vi "FRCts20_Backend_SaveTimer.vi"(8 "error in (no error)":errorcluster, 10 "Data Changed?":bool) -> (0 "error out":errorcluster)   [LabVIEW 2014, in "FRCts20_Backend_Engine.lvlib"]
doc: "This counts the time and if we have reached 5 minutes of idle time and the data changed, we send an AMC command to save everything."
uses:
  FRCts20_Backend_Engine.lvlib
  FRCts20_Backend_FGVOperation.ctl
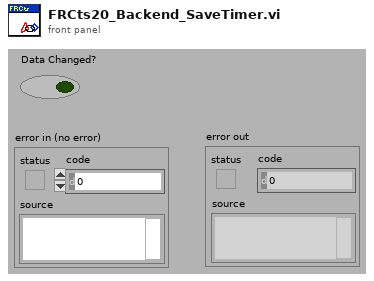
[diagram p1: front panel]
types:
  T1 = typedef "FRCts20_Backend_Engine.lvlib/FRCts20_Backend_FGVOperation.ctl" = enum16{"Initialize", "EnqueueMessage", "EnqueueDataReturn", "FlushMessage", "FlushDataReturn"}
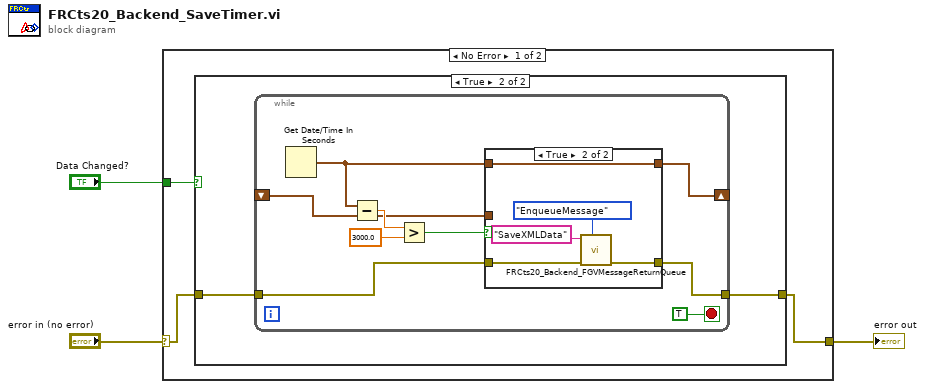
[diagram p0: block diagram]
diagram:
  n1 = case shown="No Error" "error in (no error)" {
    selector: "error in (no error)" -> [w5 w26]
    tunnel: [w4 w26] -> w2
    tunnel: "Data Changed?" -> [w6 _]
    frame No Error {
      n2 = case shown="True" w6 {
        tunnel: w5 -> [w7 w9]
        tunnel: [w7 w8] -> w4
        frame False {
        }
        frame True {
          n3 = while {
            shift-right: [w11] -> _
            shift-left: _ -> [w10]
            tunnel: w9 -> [w14]
            tunnel: [w13] -> w8
            stop <- TRUE stop-if-true
            n4 = Get Date/Time In Seconds() -> (seconds since 1Jan1904=w12:timestamp)
            n5 = Subtract(x=w12, y=w10) -> (x-y=w17:dbl)
            n6 = Greater?(x=w17, y=3000.0) -> (0:w15:bool)
            n7 = case shown="True" w15 {
              tunnel: w14 -> [w20 w23]
              tunnel: [w20 w22] -> w13
              tunnel: w12 -> [_ w21]
              tunnel: [w19 w21] -> w11
              tunnel: w10 -> [w19 _]
              frame False {
              }
              frame True {
                n8 = call "FRCts20_Backend_FGVMessageReturnQueue.vi"("Operation"=FRCts20_Backend_FGVOperation."EnqueueMessage", "error in (no error)"=w23, "Message Name"="SaveXMLData") -> ("error out"=w22:errorcluster)  [unwired: 7 in, 1 out]
              }
            }
          }
        }
      }
    }
    frame Error {
    }
  }
  "error out" <- w2
